vi "init_proc_img_Q.vi"() -> (8 "Proc Img Notifier Out":T1)   [LabVIEW 2023]
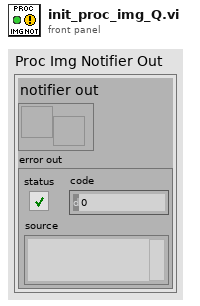
[diagram p1: front panel]
types:
  T1 = cluster{"notifier out":refnum<notifier>, "error out":errorcluster}
  T2 = cluster{"A Counts":i32, "A Counts / 5F":dbl, "Update Counts?":bool, "Actual Width":u32, "B Counts / 5F ":dbl, "B Counts":i32, "Actual Height":u32, "Accumulated Image ":i16[][], "Total Counts":i32, "B Array i02":sgl[][], "A Array i01":sgl[][], "B Array":i16[][], "A Array":i16[][], "Region of interest":i32[], "Count Buffer Size 1":i32, "Init Img":i16[][], "counts /F":i16}
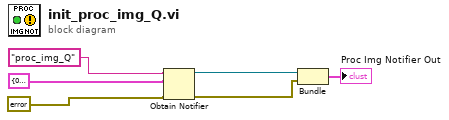
[diagram p0: block diagram]
diagram:
  n1 = Obtain Notifier(name (unnamed)="proc_img_Q", notification data type=T2 {"A Counts"=0, "A Counts / 5F"=0.0, "Update Counts?"=FALSE, "Actual Width"=0, "B Counts / 5F "=0.0, "B Counts"=0, "Actual Height"=0, "Accumulated Image "=[], "Total Counts"=0, "B Array i02"=[], "A Array i01"=[], "B Array"=[], "A Array"=[], "Region of interest"=[0, 0, 1020, 1020], "Count Buffer Size 1"=2000000, "Init Img"=[], "counts /F"=0}, error in (no error)=errorcluster {"status"=FALSE, "code"=0, "source"=""}) -> (notifier out=w3:refnum<notifier>, error out=w2:errorcluster)  [unwired: 1 in, 1 out]
  n2 = Bundle("notifier out"=w3, "error out"=w2) -> (→"Proc Img Notifier Out":T1)  [unwired: 1 in]
